vi "Add Channel to Sequence.vi"(8 "error in (no error)":errorcluster, 11 "UI in":refnum<class "UI.lvclass">) -> (0 "error out":errorcluster, 3 "UI out":refnum<class "UI.lvclass">)   [LabVIEW 2015, in "UI.lvlib" / "UI.lvclass"]
uses:
  UI.lvclass
  UI.lvclass/UI.ctl
  Sequencer/Sequencer Messages/Insert Channel Msg/Insert Channel Msg.lvclass
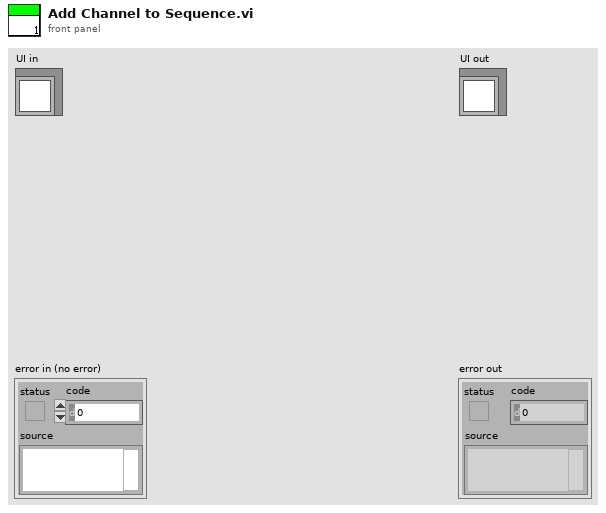
[diagram p1: front panel]
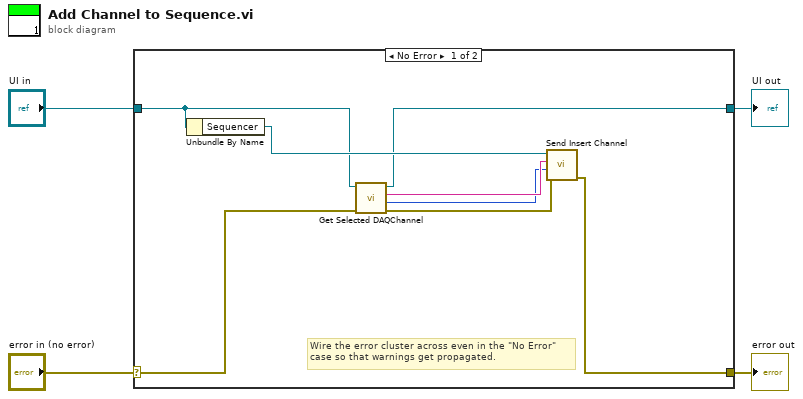
[diagram p0: block diagram]
diagram:
  n1 = case shown="No Error" "error in (no error)" {
    selector: "error in (no error)" -> [w7 w14]
    tunnel: [w6 w14] -> w3
    tunnel: [w10 w13] -> w1
    tunnel: "UI in" -> [w11 w13]
    frame No Error {
      # "Wire the error cluster across even in the \"No Error\"\ncase so that warnings get propagated."
      n2 = Unbundle By Name(w11) -> ("Sequencer"=w12:refnum<class "Message Enqueuer.lvclass">)
      n3 = call "Get Selected DAQChannel.vi"("error in (no error)"=w7, "UI in"=w11) -> ("error out"=w8:errorcluster, "Type"=w5:enum16{"AO", "DO", "AI"}, "Channel Out"=w9:tag, "UI out"=w10:refnum<class "UI.lvclass">)  [unwired: 6 in]
      n4 = call "Send Insert Channel.vi"("error in (no error)"=w8, "ChannelType"=w5, "Device Address"=w9, "Message Enqueuer in"=w12) -> ("error out"=w6:errorcluster)  [unwired: 6 in, 1 out]
    }
    frame Error {
    }
  }
  "error out" <- w3
  "UI out" <- w1
